vi "Inst.KH7008.AppLauncher.vi"(8 "error in":errorcluster, 11 "Debug Mode":bool) -> (0 "error out":errorcluster)   [LabVIEW 2019, in "Inst.KH7008.lvlib" / "Inst.Krohn-Hite-7008.lvclass"]
uses:
  Inst.Krohn-Hite-7008.lvclass
  Inst UI.Krohn-Hite-7008/Inst UI.Krohn-Hite-7008.lvclass
  <userlib>/LevyLab/Instrument Framework/Instrument/Instrument.lvclass
  <userlib>/LevyLab/Instrument Framework/Instrument UI/Instrument UI.lvclass
  <vilib>/JKI/JKI SMO/SMO/Typedefs/SMOState --Enum.ctl
  <vilib>/JKI/JKI SMO/SMO/SMO.lvclass
  <vilib>/JKI/JKI SMO/SMO.UI/SMO.UI.lvclass
  C:/Program Files/National Instruments/LabVIEW 2019/user.lib/LevyLab/Instrument Framework/Instrument Types/Amplifier/Instrument.Amplifier.lvclass
  C:/Program Files/National Instruments/LabVIEW 2019/user.lib/LevyLab/Instrument Framework/Instrument/Instrument.lvclass
  C:/Program Files/National Instruments/LabVIEW 2019/vi.lib/JKI/JKI SMO/SMO/SMO.lvclass
  C:/Program Files/National Instruments/LabVIEW 2019/user.lib/LevyLab/Instrument Framework/Instrument UI/Instrument UI.lvclass
  C:/Program Files/National Instruments/LabVIEW 2019/vi.lib/JKI/JKI SMO/SMO.UI/SMO.UI.lvclass
panel:
  in  "Examine Configuration.ini":bool
  in  "Splash Status":string="Push Start to Start..." caption="String"
  in  "Start Application":bool caption="Play"
  in  "Stop Application":bool caption="Stop"
  out "SMO State":T1
  # "Example Instrument SMO Test Launcher"
  # "For instructions on how to use the JKI State Machine Objects, examples and video tutorials, visit:\nhttp://jki.net/state-machine-objects/\n\nJKI State Machine Objects™\nhttp://jki.net/state-machine-objects/\nCopyright (C) 2005-2015, JKI <info@jki.net>\nALL RIGHTS RESERVED"
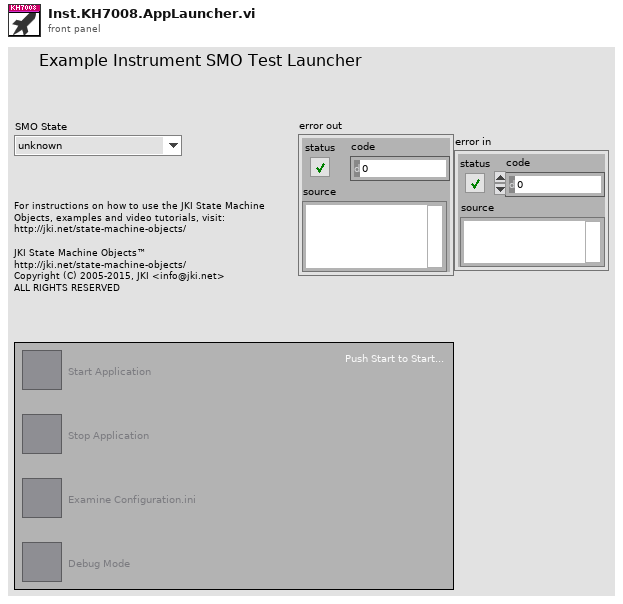
[diagram p1: front panel]
types:
  T1 = typedef "SMO.lvclass/SMOState --Enum.ctl" = enum16{"unknown", "Created", "Started", "Stopped"}
  T2 = enum32{"Invalid", "Standard", "Closed", "Hidden", "Minimized", "Maximized"}
  T3 = enum32{"invalid app kind", "Development System", "Run Time System", "Student Edition", "Embedded LabVIEW", "Evaluation", "Custom"}
  T4 = cluster{"Core":cluster{"Current VI Reference":refnum<vi>, "Close Panel on Exit?":bool}, "Instruments":refnum<class "Inst.Krohn-Hite-7008.lvclass">[], "Instrument UI":refnum<class "Inst UI.Krohn-Hite-7008.lvclass">[]}
  T5 = cluster{"Current VI Reference":refnum<vi>, "Close Panel on Exit?":bool}
  T6 = typedef "SMO.lvclass/Public Events.ctl" = cluster{"Error":refnum<user-event>, "State":refnum<user-event>, "Reserve State":refnum<user-event>}
  T7 = cluster{"Event Registration Refnum":refnum<event-registration>}
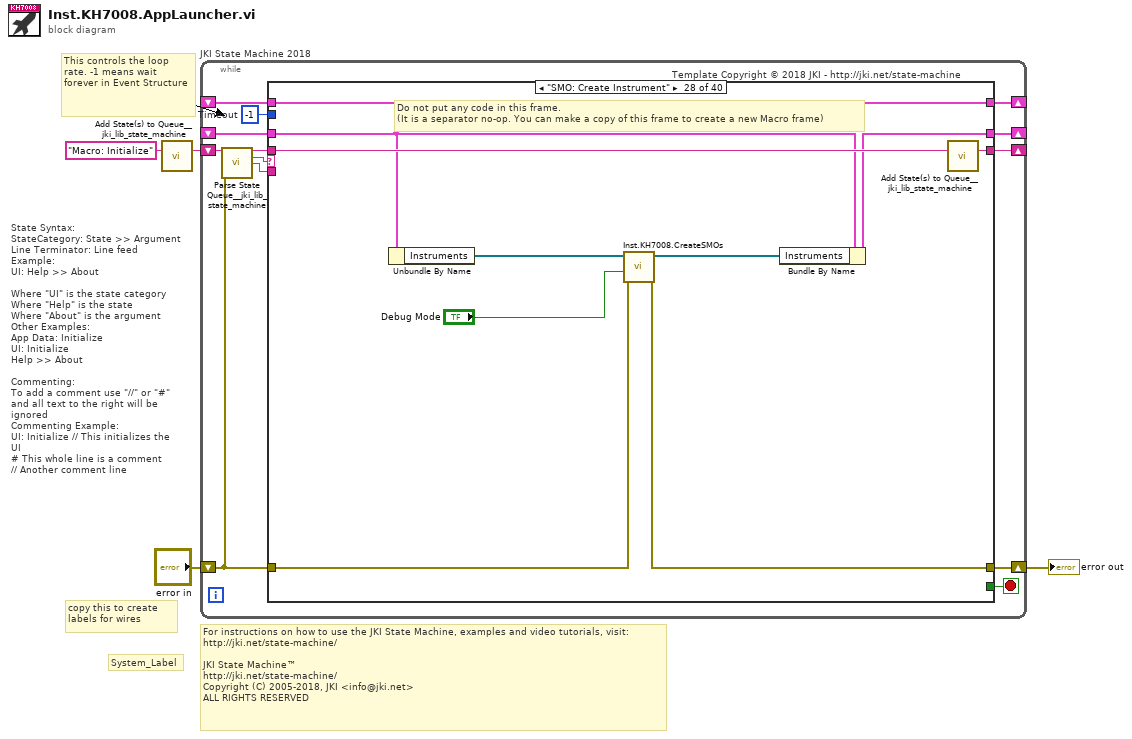
[diagram p0: block diagram]
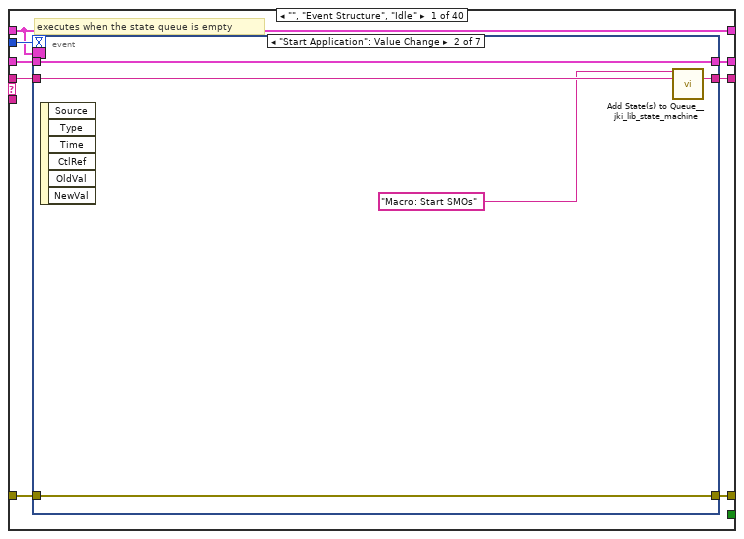
[diagram p2: hidden frame]
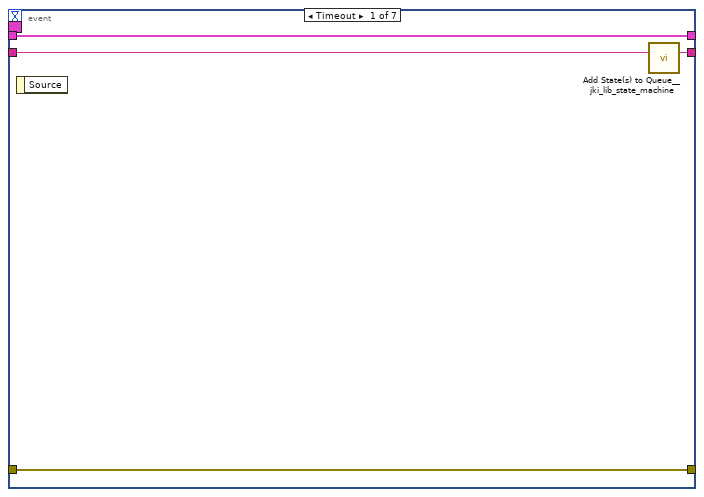
[diagram p3: hidden frame]
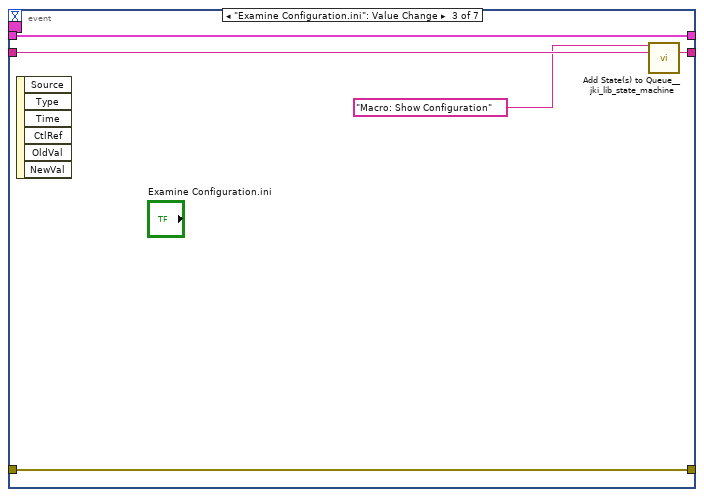
[diagram p4: hidden frame]
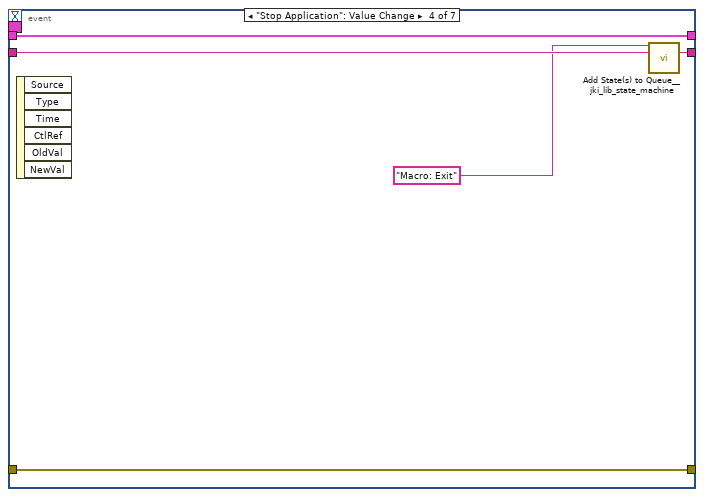
[diagram p5: hidden frame]
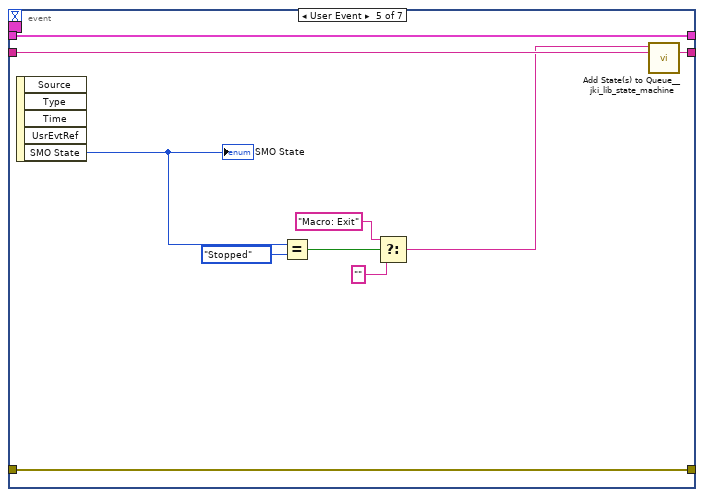
[diagram p6: hidden frame]
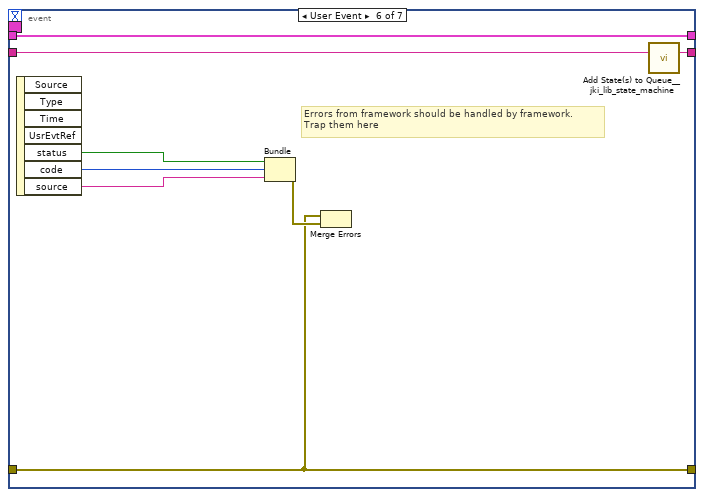
[diagram p7: hidden frame]
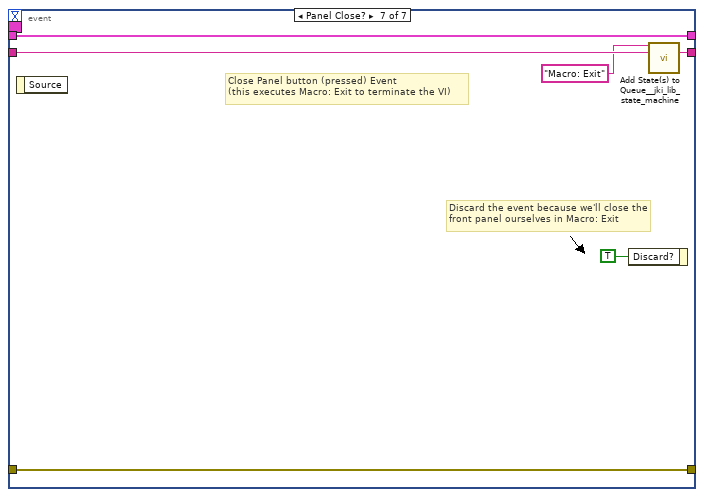
[diagram p8: hidden frame]
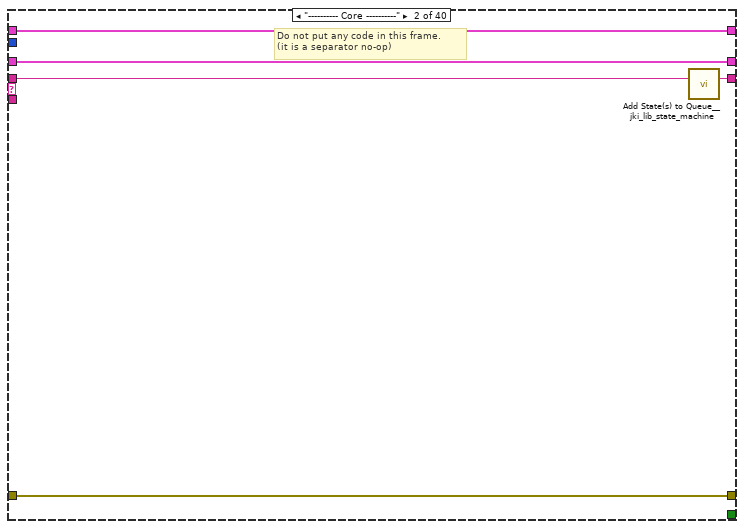
[diagram p9: hidden frame]
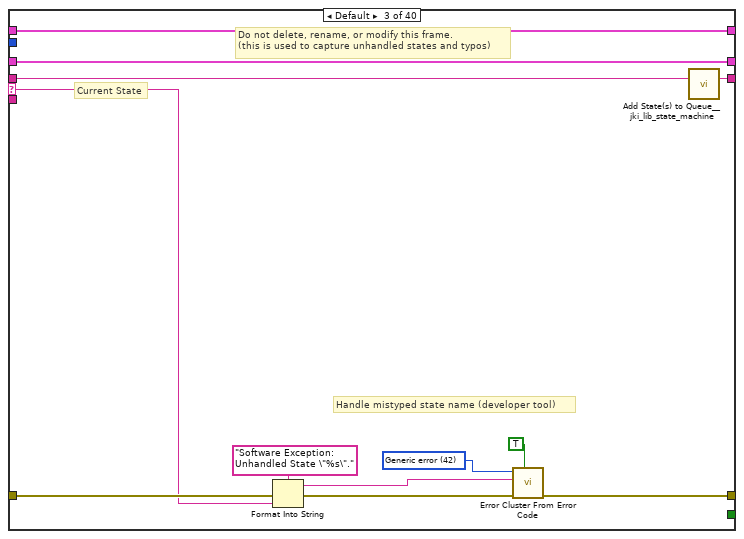
[diagram p10: hidden frame]
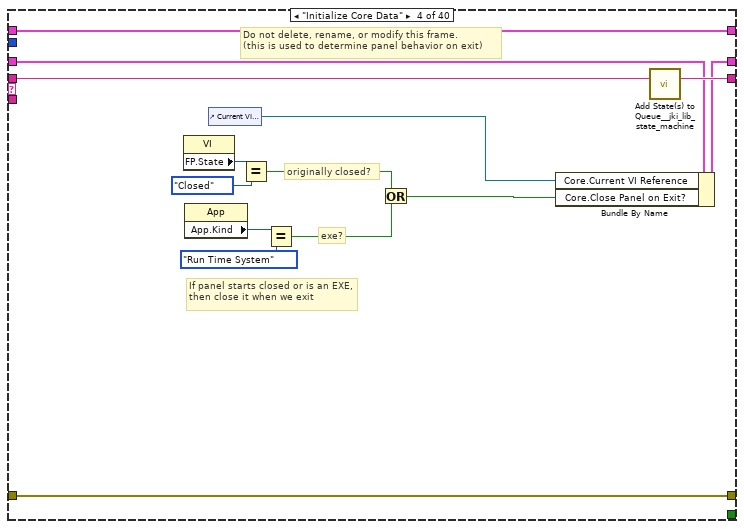
[diagram p11: hidden frame]
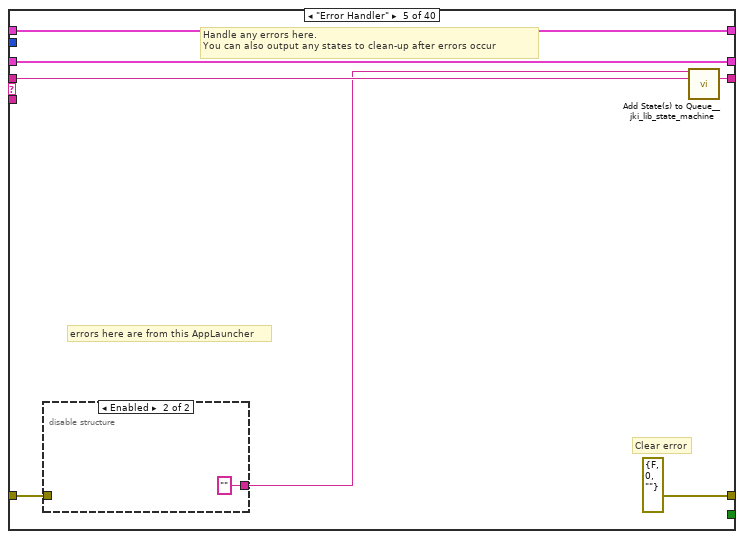
[diagram p12: hidden frame]
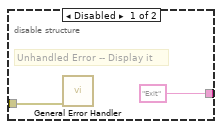
[diagram p13: hidden frame]
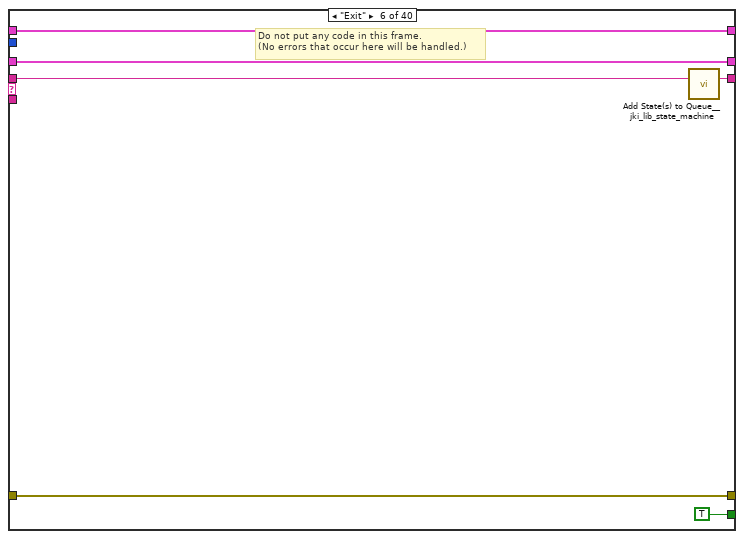
[diagram p14: hidden frame]
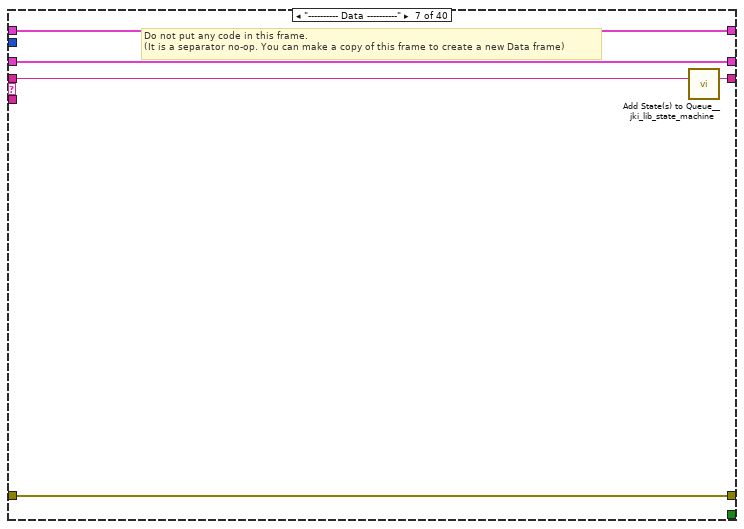
[diagram p15: hidden frame]
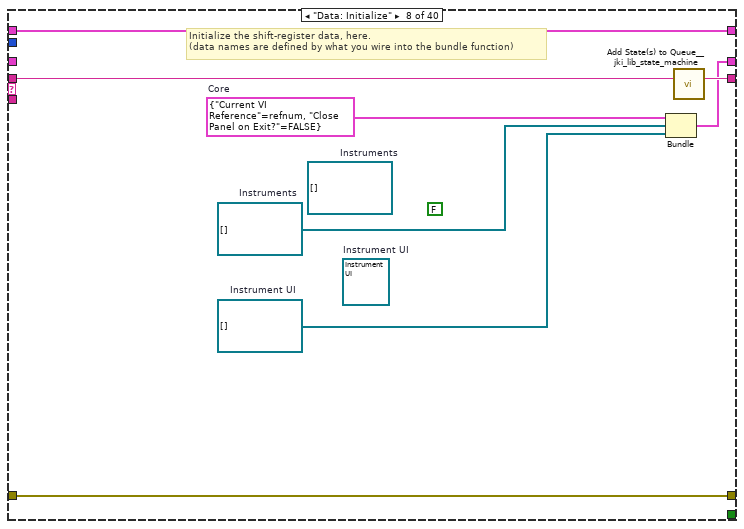
[diagram p16: hidden frame]
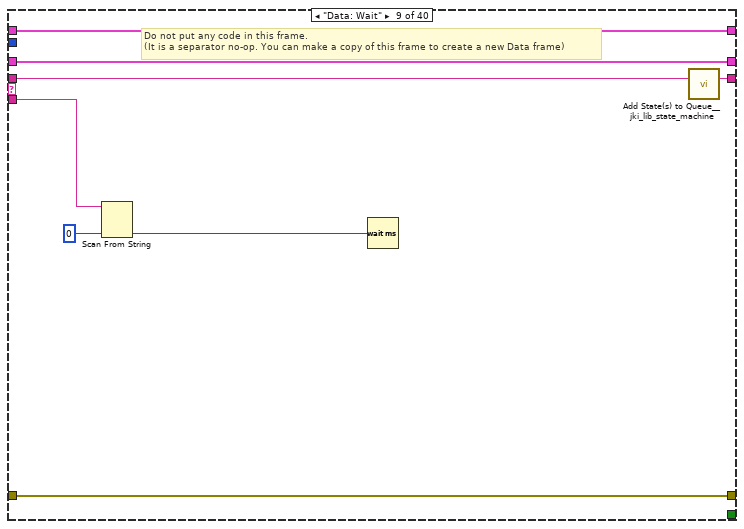
[diagram p17: hidden frame]
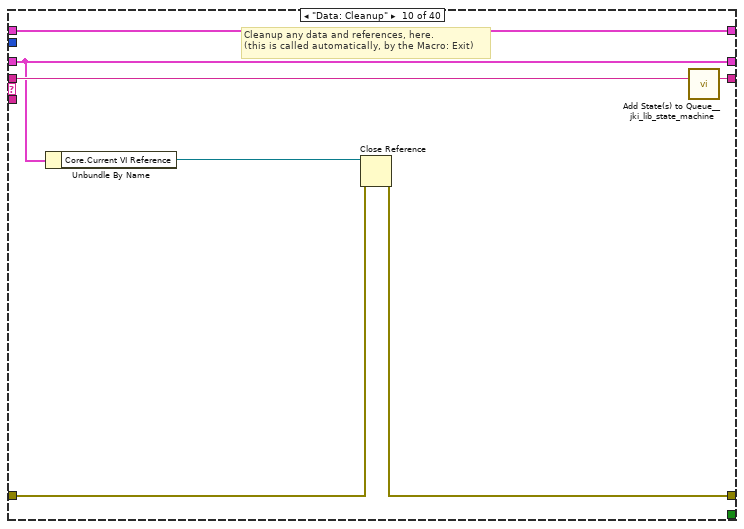
[diagram p18: hidden frame]
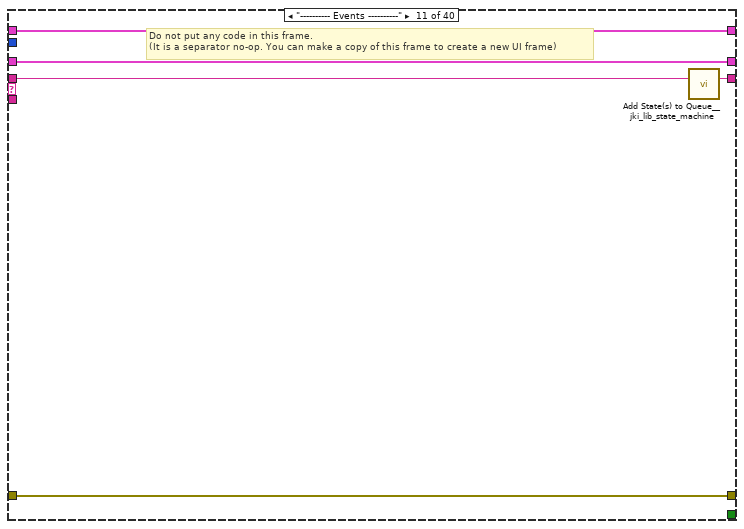
[diagram p19: hidden frame]
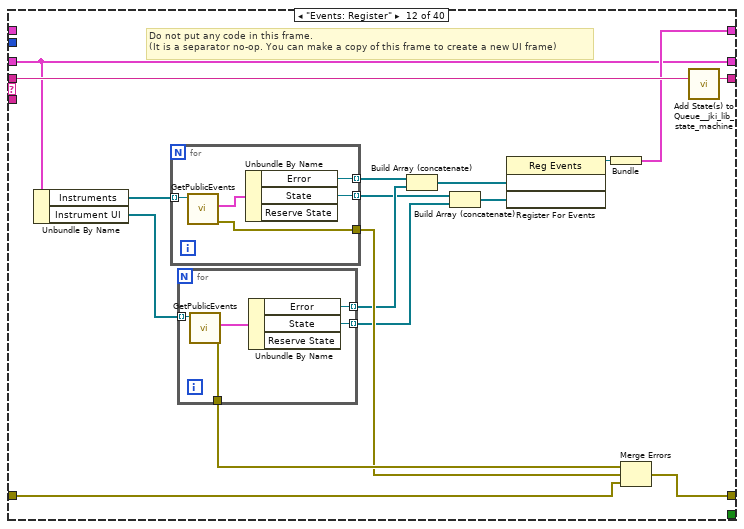
[diagram p20: hidden frame]
diagram:
  # "For instructions on how to use the JKI State Machine, examples and video tutorials, visit:\nhttp://jki.net/state-machine/\n\nJKI State Machine™\nhttp://jki.net/state-machine/\nCopyright (C) 2005-2018, JKI <info@jki.net>\nALL RIGHTS RESERVED"
  # "State Syntax:\nStateCategory: State >> Argument\nLine Terminator: Line feed\nExample:\nUI: Help >> About\n\nWhere \"UI\" is the state category\nWhere \"Help\" is the state\nWhere \"About\" is the argument\nOther Examples:\nApp Data: Initialize\nUI: Initialize\nHelp >> About\n\nCommenting:\nTo add a comment use \"//\" or \"#\" and all text to the right will be ignored\nCommenting Example:\nUI: Initialize // This initializes the UI\n# This whole line is a comment\n// Another comment line"
  # "copy this to create labels for wires"
  # "This controls the loop rate. -1 means wait forever in Event Structure"
  # "System_Label"
  n1 = call <vilib>:"Add State(s) to Queue__jki_lib_state_machine.vi"("State(s) in (\"\")"="Macro: Initialize") -> ("States Out"=w4:string)  [unwired: 14 in]
  n2 = while "JKI State Machine 2018" {
    shift-right: [w11] -> _
    shift-left: _ -> [w6]
    shift-right: [w14] -> w2
    shift-left: "error in" -> [w9]
    shift-right: [w13] -> _
    shift-left: w4 -> [w15]
    shift-right: [w8] -> _
    shift-left: _ -> [w7]
    stop <- w12 stop-if-true
    w10 = -1  # Timeout
    # "Template Copyright © 2018 JKI - http://jki.net/state-machine"
    n3 = call <vilib>:"Parse State Queue__jki_lib_state_machine.vi"("State Queue"=w15, "Error In (no error)"=w9) -> ("Remaining States"=w17:string, "Current State"=w5:string, "Arguments"=w16:string)  [unwired: 11 in]
    n4 = case shown="\"SMO: Create Instrument\"" w5 {
      selector: w5 -> [_ _ w75 _ _ _ _ _ _ _ _ _ _ _ _ _ _ _ _ _ _ _ _ _ _ _ _ _ _ _ _ _ _ _ _ _ _ _ _ _]
      tunnel: w17 -> [w25 w73 w79 w99 w106 w115 w120 w128 w136 w143 w148 w165 w181 w186 w193 w200 w212 w290 w297 w305 w310 w316 w322 w328 w334 w346 w351 w361 w370 w385 w397 w407 w425 w443 w461 w479 w497 w513 w520 w525]
      tunnel: w16 -> [_ _ _ _ _ _ _ _ w131 _ _ _ _ _ _ w195 w206 _ _ _ _ _ _ _ _ _ _ _ _ _ _ _ _ _ _ _ _ _ w517 _]
      tunnel: [w22 w71 w81 w96 errorcluster {"status"=FALSE, "code"=0, "source"=""} ("error out") w112 w118 w123 w134 w139 w146 w158 w177 w184 w188 w196 w209 w280 w294 w303 w308 w314 w320 w326 w332 w344 w349 w353 w362 w378 w391 w403 w421 w439 w458 w476 w494 w511 w515 w523] -> w14
      tunnel: w9 -> [w21 w71 w80 w96 w102 w112 w118 w123 w134 w140 w146 w157 w178 w184 w190 w197 w210 w281 w292 w303 w308 w314 w320 w326 w332 w344 w349 w354 w363 w379 w392 w402 w420 w438 w456 w474 w492 w511 w516 w523]
      tunnel: [w24 w72 w78 w98 w105 w114 w119 w127 w135 w142 w147 w164 w180 w185 w192 w199 w211 w289 w296 w304 w309 w315 w321 w327 w333 w345 w350 w360 w369 w384 w396 w406 w424 w442 w460 w478 w496 w512 w519 w524] -> w13
      tunnel: [_ _ _ _ _ TRUE _ _ _ _ _ _ _ _ _ _ _ _ _ _ _ _ _ _ _ _ _ _ _ _ _ _ _ _ _ _ _ _ _ _] -> w12
      tunnel: [w20 w70 w77 w97 w103 w113 w117 w126 w133 w138 w145 w162 w179 w183 w191 w198 w208 w278 w293 w302 w307 w313 w319 w325 w331 w343 w348 w358 w365 w381 w394 w404 w422 w440 w457 w475 w493 w510 w518 w522] -> w11
      tunnel: w10 -> [w19 _ _ _ _ _ _ _ _ _ _ _ _ _ _ _ _ _ _ _ _ _ _ _ _ _ _ _ _ _ _ _ _ _ _ _ _ _ _ _]
      tunnel: [w18 w69 w74 w86 w101 w110 w116 w124 w132 w137 w144 w163 w176 w182 w189 w194 w205 w279 w295 w301 w306 w311 w317 w324 w330 w337 w347 w359 w368 w383 w395 w405 w423 w441 w459 w477 w495 w509 w514 w521] -> w8
      tunnel: w7 -> [w18 w69 w74 w86 w101 w110 w116 w124 w132 w137 w144 _ w176 w182 w189 w194 w205 w279 w295 w301 w306 w311 w317 w324 w330 w337 w347 w359 w368 w383 w395 w405 w423 w441 w459 w477 w495 w509 w514 w521]
      tunnel: w6 -> [w23 w70 w77 w92 w103 w113 w117 _ w133 w138 w145 w162 w179 w183 w191 w198 w208 w278 w293 w302 w307 w313 w319 w325 w331 w343 w348 w356 w366 w382 w394 w404 w422 w440 w457 w475 w493 w510 w518 w522]
      frame "", "Event Structure", "Idle" {
        # "executes when the state queue is empty"
        n5 = event shown="[1] \"Start Application\": Value Change" {
          selector: w18 -> [_ _ _ _ _ _ _]
          dyn-events: _ -> [_ _ _ _ _ _ _]
          timeout: w19 -> [_ _ _ _ _ _ _]
          tunnel: w25 -> [w29 w34 w39 w44 w54 w62 w68]
          tunnel: [w28 w33 w38 w43 w53 w61 w67] -> w24
          tunnel: w23 -> [w26 w31 w36 w41 w51 w60 w65]
          tunnel: [w27 w32 w37 w42 w52 w55 w66] -> w22
          tunnel: w21 -> [w27 w32 w37 w42 w52 w55 w66]
          tunnel: [w26 w31 w36 w41 w51 w60 w65] -> w20
          event Timeout {
            n6 = event-data() -> ()  [unwired: 1 in, 1 out]
            n7 = call <vilib>:"Add State(s) to Queue__jki_lib_state_machine.vi"("State(s) in (\"\")"=w29) -> ("States Out"=w28:string)  [unwired: 14 in]
          }
          event "Start Application": Value Change {
            n8 = event-data() -> ()  [unwired: 1 in, 6 out]
            n9 = call <vilib>:"Add State(s) to Queue__jki_lib_state_machine.vi"("State(s) in Front (\"\")"="Macro: Start SMOs" ("State(s) in Front (\"\")"), "State(s) in (\"\")"=w34) -> ("States Out"=w33:string)  [unwired: 13 in]
          }
          event "Examine Configuration.ini": Value Change {
            n10 = event-data() -> ()  [unwired: 1 in, 6 out]
            n11 = call <vilib>:"Add State(s) to Queue__jki_lib_state_machine.vi"("State(s) in Front (\"\")"="Macro: Show Configuration" ("State(s) in Front (\"\")"), "State(s) in (\"\")"=w39) -> ("States Out"=w38:string)  [unwired: 13 in]
          }
          event "Stop Application": Value Change {
            n12 = event-data() -> ()  [unwired: 1 in, 6 out]
            n13 = call <vilib>:"Add State(s) to Queue__jki_lib_state_machine.vi"("State(s) in Front (\"\")"="Macro: Exit" ("State(s) in Front (\"\")"), "State(s) in (\"\")"=w44) -> ("States Out"=w43:string)  [unwired: 13 in]
          }
          event User Event {
            n14 = event-data() -> ("SMO State"=w46:T1)  [unwired: 1 in, 4 out]
            "SMO State" <- w46
            n15 = Equal?(x=w46, y=SMOState_--Enum."Stopped") -> (x = y?=w49:bool)
            n16 = Select(t="Macro: Exit", s=w49, f="" ("State(s) in Front (\"\")")) -> (s? t:f=w45:string)
            n17 = call <vilib>:"Add State(s) to Queue__jki_lib_state_machine.vi"("State(s) in Front (\"\")"=w45, "State(s) in (\"\")"=w54) -> ("States Out"=w53:string)  [unwired: 13 in]
          }
          event User Event {
            # "Errors from framework should be handled by framework.\nTrap them here"
            n18 = event-data() -> ("status"=w56:bool, "code"=w58:i32, "source"=w57:string)  [unwired: 1 in, 4 out]
            n19 = Bundle("status"=w56, "code"=w58, "source"=w57) -> (w59:errorcluster)  [unwired: 1 in]
            n20 = Merge Errors(w55, w59) -> ()  [unwired: 1 out]
            n21 = call <vilib>:"Add State(s) to Queue__jki_lib_state_machine.vi"("State(s) in (\"\")"=w62) -> ("States Out"=w61:string)  [unwired: 14 in]
          }
          event Panel Close? {
            # "Discard the event because we'll close the front panel ourselves in Macro: Exit"
            # "Close Panel button (pressed) Event\n(this executes Macro: Exit to terminate the VI)"
            n22 = event-data() -> ()  [unwired: 1 in, 1 out]
            n23 = event-data("Discard?"=TRUE) -> ()  [unwired: 1 in, 1 out]
            n24 = call <vilib>:"Add State(s) to Queue__jki_lib_state_machine.vi"("State(s) in Front (\"\")"="Macro: Exit", "State(s) in (\"\")"=w68) -> ("States Out"=w67:string)  [unwired: 13 in]
          }
        }
      }
      frame "---------- Core ----------" {
        # "Do not put any code in this frame.\n(it is a separator no-op)"
        n25 = call <vilib>:"Add State(s) to Queue__jki_lib_state_machine.vi"("State(s) in (\"\")"=w73) -> ("States Out"=w72:string)  [unwired: 14 in]
      }
      frame Default {
        w84 = 42 items=["No error", "Argument error", "Memory is full", "Out of zone", "End of file", "File already open", "Generic file I/O error", "File not found", "File permission error", "Disk is full", "Duplicate path", "Too many files open", "System feature not enabled", "Resource file not found", "Cannot add resource", "Resource not found", "Image not found", "Image memory error", "Pen does not exist", "Config type invalid", "Config token not found", "Config parse error", "Config memory error", "Bad external code format", "Bad external code offset", "External code not present", "Null window", "Destroy window error", "Null menu", "Print aborted", "Bad print record", "Print driver error", "Windows error during printing", "Memory error during printing", "Print dialog error", "Generic print error", "Invalid device refnum", "Device not found", "Device parameter error", "Device unit error", "Cannot open device", "Device call aborted", "Generic error", "Cancelled by user", "Object ID too low", "Object ID too high", "Object not in heap", "Unknown heap", "Unknown object (invalid DefProc)", "Unknown object (DefProc not in table)", "Message out of range", "Invalid (null) method", "Unknown message", "Manager call not supported", "Bad address", "Network operation in progress", "Network operation timed out", "Connection is busy", "Network attribute not supported", "Network error", "Address in use", "System out of memory", "Connection aborted", "Connection refused", "Not connected", "Already connected", "Connection closed", "Initialization error (interapplication manager)", "Bad occurrence", "Wait on unbound occurrence handler", "Occurrence queue overflow", "Datalog type conflict", "Unused", "Unrecognized type (interapplication manager)", "Memory corrupt", "Failed to make temporary DLL", "Old CIN version", "Drag socket not found", "Failed to load drop-object", "Failed to register OLE object", "Failed to release OLE object", "Format specifier type mismatch", "Unknown format specifier", "Too few format specifiers", "Too many format specifiers", "Scan failed", "Newer CIN version", "Error converting to variant", "Runtime menu error", "Password tampered", "Variant attribute not found", "Incompatible variant data type", "Event data is not available", "Event Store is not present", "Occurrence is not found", "Event Queue is not created", "Event info is not available", "Refnum passed is NULL", "Error retrieving Class GUID", "Error retrieving CoClass GUID", "Error retrieving TypeLib GUID.", "Bad built application magic bytes.", "Specific driver is different from the specific driver associated with the Logical Name.", "There is no session opened to the class driver.", "Max Error", "MAX - Error with config objects", "MAX - Error loading configuration", "MAX - Group not supported"]
        # "Current State"
        # "Do not delete, rename, or modify this frame.\n(this is used to capture unhandled states and typos)"
        # "Handle mistyped state name (developer tool)"
        n26 = Format Into String(format string="Software Exception: Unhandled State \"%s\"." ("message"), error in=w80, w75) -> (resulting string=w83:string, error out=w82:errorcluster)  [unwired: 1 in]
        n27 = call <vilib>:"Error Cluster From Error Code.vi"("show call chain? (False)"=TRUE, "error in (no error)"=w82, "error message (\"\")"=w83, "error code (0)"=w84) -> ("error out"=w81:errorcluster)  [unwired: 5 in]
        n28 = call <vilib>:"Add State(s) to Queue__jki_lib_state_machine.vi"("State(s) in (\"\")"=w79) -> ("States Out"=w78:string)  [unwired: 14 in]
      }
      frame "Initialize Core Data" {
        # "Do not delete, rename, or modify this frame.\n(this is used to determine panel behavior on exit)"
        # "originally closed?"
        # "exe?"
        # "If panel starts closed or is an EXE, then close it when we exit"
        n29 = property class="VI"() -> ("FP.State"=w89:T2)  [unwired: 2 in, 2 out]
        n30 = property class="App"() -> ("App.Kind"=w95:T3)  [unwired: 2 in, 2 out]
        n31 = control-ref of="Current VI Reference"() -> (w90:refnum<vi>)
        n32 = Equal?(x=w89, y=T2."Closed" ("Front Panel Window:State")) -> (x = y?=w87:bool)
        n33 = Equal?(x=w95, y=T3."Run Time System" ("Application:Kind")) -> (x = y?=w93:bool)
        n34 = Or(x=w87, y=w93) -> (x .or. y?=w91:bool)
        n35 = Bundle By Name(cluster=w92, "Core.Current VI Reference"=w90, "Core.Close Panel on Exit?"=w91) -> (w97:T4)
        n36 = call <vilib>:"Add State(s) to Queue__jki_lib_state_machine.vi"("State(s) in (\"\")"=w99) -> ("States Out"=w98:string)  [unwired: 14 in]
      }
      frame "Error Handler" {
        # "errors here are from this AppLauncher"
        # "Handle any errors here.\nYou can also output any states to clean-up after errors occur"
        # "Clear error"
        n37 = disable-structure shown="Enabled" {
          disable-tunnel: w102 -> [w108 _]
          disable-tunnel: ["Exit" "" ("State(s) in Front (\"\")")] -> w100
          frame Disabled {
            # "Unhandled Error -- Display it"
            n38 = call <vilib>:"General Error Handler.vi"("error in (no error)"=w108) -> ()  [unwired: 10 in, 5 out]
          }
          frame Enabled {
          }
        }
        n39 = call <vilib>:"Add State(s) to Queue__jki_lib_state_machine.vi"("State(s) in Front (\"\")"=w100, "State(s) in (\"\")"=w106) -> ("States Out"=w105:string)  [unwired: 13 in]
      }
      frame "Exit" {
        # "Do not put any code in this frame.\n(No errors that occur here will be handled.)"
        n40 = call <vilib>:"Add State(s) to Queue__jki_lib_state_machine.vi"("State(s) in (\"\")"=w115) -> ("States Out"=w114:string)  [unwired: 14 in]
      }
      frame "---------- Data ----------" {
        # "Do not put any code in this frame.\n(It is a separator no-op. You can make a copy of this frame to create a new Data frame)"
        n41 = call <vilib>:"Add State(s) to Queue__jki_lib_state_machine.vi"("State(s) in (\"\")"=w120) -> ("States Out"=w119:string)  [unwired: 14 in]
      }
      frame "Data: Initialize" {
        (unwired) FALSE ("s")
        w122 = refnum<class "Inst.Krohn-Hite-7008.lvclass">[] []  # Instruments
        w121 = refnum<class "Inst UI.Krohn-Hite-7008.lvclass">[] []  # Instrument UI
        (unwired) refnum<class "Instrument UI.lvclass"> refnum  # Instrument UI
        (unwired) refnum<class "Instrument.lvclass">[] []  # Instruments
        w125 = T5 {"Current VI Reference"=refnum, "Close Panel on Exit?"=FALSE}  # Core
        # "Initialize the shift-register data, here.\n(data names are defined by what you wire into the bundle function)"
        n42 = Bundle("Core"=w125, "Instruments"=w122, "Instrument UI"=w121) -> (w126:T4)  [unwired: 1 in]
        n43 = call <vilib>:"Add State(s) to Queue__jki_lib_state_machine.vi"("State(s) in (\"\")"=w128) -> ("States Out"=w127:string)  [unwired: 14 in]
      }
      frame "Data: Wait" {
        # "Do not put any code in this frame.\n(It is a separator no-op. You can make a copy of this frame to create a new Data frame)"
        n44 = Scan From String(input string=w131, default 1=u32 0) -> (output 1=w129:u32)  [unwired: 3 in, 3 out]
        n45 = Wait (ms)(milliseconds to wait=w129) -> ()  [unwired: 1 out]
        n46 = call <vilib>:"Add State(s) to Queue__jki_lib_state_machine.vi"("State(s) in (\"\")"=w136) -> ("States Out"=w135:string)  [unwired: 14 in]
      }
      frame "Data: Cleanup" {
        # "Cleanup any data and references, here.\n(this is called automatically, by the Macro: Exit)"
        n47 = Unbundle By Name(w138) -> ("Core.Current VI Reference"=w141:refnum<vi>)
        n48 = Close Reference(reference=w141, error in (no error)=w140) -> (error out=w139:errorcluster)
        n49 = call <vilib>:"Add State(s) to Queue__jki_lib_state_machine.vi"("State(s) in (\"\")"=w143) -> ("States Out"=w142:string)  [unwired: 14 in]
      }
      frame "---------- Events ----------" {
        # "Do not put any code in this frame.\n(It is a separator no-op. You can make a copy of this frame to create a new UI frame)"
        n50 = call <vilib>:"Add State(s) to Queue__jki_lib_state_machine.vi"("State(s) in (\"\")"=w148) -> ("States Out"=w147:string)  [unwired: 14 in]
      }
      frame "Events: Register" {
        # "Do not put any code in this frame.\n(It is a separator no-op. You can make a copy of this frame to create a new UI frame)"
        n51 = Unbundle By Name(w162) -> ("Instruments"=w161:refnum<class "Inst.Krohn-Hite-7008.lvclass">[], "Instrument UI"=w160:refnum<class "Inst UI.Krohn-Hite-7008.lvclass">[])
        n52 = for {
          tunnel: w161 -> [w175] mode=indexing
          tunnel: [w174] -> w155
          tunnel: [w172] -> w154 mode=indexing
          tunnel: [w171] -> w151 mode=indexing
          n53 = call <vilib>:"GetPublicEvents.vi"("SMO"=w175) -> ("error out"=w174:errorcluster, "Public Events"=w173:T6)  [unwired: 8 in, 1 out]
          n54 = Unbundle By Name(w173) -> ("Error"=w172:refnum<user-event>, "State"=w171:refnum<user-event>)  [unwired: 1 out]
        }
        n55 = for {
          tunnel: w160 -> [w170] mode=indexing
          tunnel: [w169] -> w159
          tunnel: [w167] -> w153 mode=indexing
          tunnel: [w166] -> w149 mode=indexing
          n56 = call <vilib>:"GetPublicEvents.vi"("SMO"=w170) -> ("error out"=w169:errorcluster, "Public Events"=w168:T6)  [unwired: 8 in, 1 out]
          n57 = Unbundle By Name(w168) -> ("Error"=w167:refnum<user-event>, "State"=w166:refnum<user-event>)  [unwired: 1 out]
        }
        n58 = Build Array (concatenate)(w154, w153) -> (w152:refnum<user-event>[])
        n59 = Build Array (concatenate)(w151, w149) -> (w150:refnum<user-event>[])
        n60 = register-events(w152, w150) -> (reference out=w156:refnum<event-registration>)  [unwired: 2 in, 1 out]
        n61 = Bundle("Event Registration Refnum"=w156) -> (w163:T7)  [unwired: 1 in]
        n62 = Merge Errors(w159, w155, w157) -> (w158:errorcluster)
        n63 = call <vilib>:"Add State(s) to Queue__jki_lib_state_machine.vi"("State(s) in (\"\")"=w165) -> ("States Out"=w164:string)  [unwired: 14 in]
      }
      frame "Events: Unregister" {
        # "Do not put any code in this frame.\n(It is a separator no-op. You can make a copy of this frame to create a new UI frame)"
        n64 = Unregister For Events(event registration refnum=w176, error in=w178) -> (error out=w177:errorcluster)
        n65 = call <vilib>:"Add State(s) to Queue__jki_lib_state_machine.vi"("State(s) in (\"\")"=w181) -> ("States Out"=w180:string)  [unwired: 14 in]
      }
      frame "---------- UI ----------" {
        # "Do not put any code in this frame.\n(It is a separator no-op. You can make a copy of this frame to create a new UI frame)"
        n66 = call <vilib>:"Add State(s) to Queue__jki_lib_state_machine.vi"("State(s) in (\"\")"=w186) -> ("States Out"=w185:string)  [unwired: 14 in]
      }
      frame "UI: Initialize" {
        # "Initialize the User Interface, here.\n(this is called automatically, by the Macro: Init)"
        n67 = invoke on="Stop Application" class="Bool" method="Reinit To Default"() -> ()  [unwired: 3 in, 3 out]
        n68 = invoke on="error out" class="Clust (strict)" method="Reinit To Default"() -> ()  [unwired: 3 in, 3 out]
        n69 = invoke on="SMO State" class="Enum (strict)" method="Reinit To Default"() -> ()  [unwired: 3 in, 3 out]
        n70 = invoke on="Start Application" class="Bool" method="Reinit To Default"() -> ()  [unwired: 3 in, 3 out]
        n71 = call <userlib>:"Fit VI window to Largest Dec__ogtk.vi"("error in (no error)"=w190, "border spacing (2 px)"=1) -> ("error out"=w188:errorcluster)  [unwired: 4 in, 1 out]
        n72 = call <vilib>:"Add State(s) to Queue__jki_lib_state_machine.vi"("State(s) in (\"\")"=w193) -> ("States Out"=w192:string)  [unwired: 14 in]
      }
      frame "UI: Cursor Set" {
        # "Argument"
        # "Set and Unset Cursor Busy.\n(Usage: \"UI: Cursor Set >> Busy|Idle\")"
        n73 = case shown="\"Busy\"" w195 {
          tunnel: w197 -> [w202 w204]
          tunnel: [w201 w203] -> w196
          frame "Idle", Default {
            n74 = call <vilib>:"Unset Busy.vi"("error in (no error)"=w202) -> ("error out"=w201:errorcluster)  [unwired: 10 in]
          }
          frame "Busy" {
            n75 = call <vilib>:"Set Busy.vi"("error in (no error)"=w204) -> ("error out"=w203:errorcluster)  [unwired: 9 in, 1 out]
          }
        }
        n76 = call <vilib>:"Add State(s) to Queue__jki_lib_state_machine.vi"("State(s) in (\"\")"=w200) -> ("States Out"=w199:string)  [unwired: 14 in]
      }
      frame "UI: Front Panel State" {
        # "Argument"
        # "Set Front Panel Open or Closed\n(Usage: \"UI: Front Panel State >> Open|Close\")"
        n77 = Unbundle By Name(w208) -> ("Core.Current VI Reference"=w207:refnum<vi>)
        n78 = case shown="\"Open\", \"Standard\", Default" w206 {
          tunnel: w210 -> [w218 w233 w244 w257 w270]
          tunnel: [w220 w234 w246 w259 w272] -> w209
          tunnel: w207 -> [w219 w231 w245 w258 w271]
          frame "Open", "Standard", Default {
            w213 = T2."Standard" ("State")
            n79 = property class="VI"(reference=w219, error in=w218) -> (reference out=w216:refnum<vi>, error out=w217:errorcluster, "FP.State"=w215:T2)
            n80 = Not Equal?(x=w215, y=w213) -> (x != y?=w214:bool)
            n81 = case shown="False" w214 {
              tunnel: [w224 w226] -> w220
              tunnel: w217 -> [w223 w226]
              tunnel: w216 -> [w222 _]
              tunnel: w213 -> [w221 _]
              frame True {
                n82 = invoke class="VI" method="FP.Open"(reference=w222, error in=w223, "Activate"=TRUE, "State"=w221) -> (error out=w224:errorcluster)  [unwired: 1 in, 4 out]
              }
              frame False {
              }
            }
          }
          frame "Close", "Closed" {
            n83 = property class="VI"(reference=w231, error in=w233) -> (reference out=w230:refnum<vi>, error out=w232:errorcluster, "FP.State"=w228:T2)
            n84 = Not Equal?(x=w228, y=T2."Closed" ("Front Panel Window:State")) -> (x != y?=w227:bool)
            n85 = case shown="True" w227 {
              tunnel: [w235 w238] -> w234
              tunnel: w232 -> [w235 w237]
              tunnel: w230 -> [_ w236]
              frame False {
              }
              frame True {
                n86 = invoke class="VI" method="FP.Close"(reference=w236, error in=w237) -> (error out=w238:errorcluster)  [unwired: 1 in, 2 out]
              }
            }
          }
          frame "Hidden", "Hide" {
            w239 = T2."Hidden" ("State")
            n87 = property class="VI"(reference=w245, error in=w244) -> (reference out=w242:refnum<vi>, error out=w243:errorcluster, "FP.State"=w241:T2)
            n88 = Not Equal?(x=w241, y=w239) -> (x != y?=w240:bool)
            n89 = case shown="True" w240 {
              tunnel: [w250 w251] -> w246
              tunnel: w243 -> [w249 w251]
              tunnel: w242 -> [w248 _]
              tunnel: w239 -> [w247 _]
              frame True {
                n90 = invoke class="VI" method="FP.Open"(reference=w248, error in=w249, "State"=w247) -> (error out=w250:errorcluster)  [unwired: 2 in, 4 out]
              }
              frame False {
              }
            }
          }
          frame "Minimize", "Minimized" {
            w252 = T2."Minimized" ("State")
            n91 = property class="VI"(reference=w258, error in=w257) -> (reference out=w255:refnum<vi>, error out=w256:errorcluster, "FP.State"=w254:T2)
            n92 = Not Equal?(x=w254, y=w252) -> (x != y?=w253:bool)
            n93 = case shown="True" w253 {
              tunnel: [w263 w264] -> w259
              tunnel: w256 -> [w262 w264]
              tunnel: w255 -> [w261 _]
              tunnel: w252 -> [w260 _]
              frame True {
                n94 = invoke class="VI" method="FP.Open"(reference=w261, error in=w262, "State"=w260) -> (error out=w263:errorcluster)  [unwired: 2 in, 4 out]
              }
              frame False {
              }
            }
          }
          frame "Maximize", "Maximized" {
            w265 = T2."Maximized" ("State")
            n95 = property class="VI"(reference=w271, error in=w270) -> (reference out=w268:refnum<vi>, error out=w269:errorcluster, "FP.State"=w267:T2)
            n96 = Not Equal?(x=w267, y=w265) -> (x != y?=w266:bool)
            n97 = case shown="True" w266 {
              tunnel: [w276 w277] -> w272
              tunnel: w269 -> [w275 w277]
              tunnel: w268 -> [w274 _]
              tunnel: w265 -> [w273 _]
              frame True {
                n98 = invoke class="VI" method="FP.Open"(reference=w274, error in=w275, "State"=w273) -> (error out=w276:errorcluster)  [unwired: 2 in, 4 out]
              }
              frame False {
              }
            }
          }
        }
        n99 = call <vilib>:"Add State(s) to Queue__jki_lib_state_machine.vi"("State(s) in (\"\")"=w212) -> ("States Out"=w211:string)  [unwired: 14 in]
      }
      frame "UI: Set Background Color" {
        # "Do not put any code in this frame.\n(It is a separator no-op. You can make a copy of this frame to create a new UI frame)"
        n100 = property class="VI"(error in=w281) -> (error out=w283:errorcluster, "Panel"=w284:refnum<vi>)  [unwired: 1 in, 1 out]
        n101 = property class="Pnl"(reference=w284, error in=w283) -> (error out=w282:errorcluster, "Panes[]"=w285:refnum<vi>[])  [unwired: 1 out]
        n102 = Index Array(array=w285, index=0) -> (element=w287:refnum<vi>)
        n103 = property class="Pane"(reference=w287, error in=w282, "PaneColor"=u32 16777238 ("Color Box")) -> (error out=w280:errorcluster)  [unwired: 1 out]
        n104 = call <vilib>:"Add State(s) to Queue__jki_lib_state_machine.vi"("State(s) in (\"\")"=w290) -> ("States Out"=w289:string)  [unwired: 14 in]
      }
      frame "UI: Open Configuration.ini" {
        # "Do not put any code in this frame.\n(It is a separator no-op. You can make a copy of this frame to create a new UI frame)"
        n105 = Unbundle By Name(w293) -> ("Instruments"=w291:refnum<class "Inst.Krohn-Hite-7008.lvclass">[])
        n106 = for {
          shift-right: [w300] -> w294
          shift-left: w292 -> [w299]
          tunnel: w291 -> [w298] mode=indexing
          n107 = call <userlib>:"Examine Configuration.vi"("error in (no error)"=w299, "Instrument in"=w298) -> ("error out"=w300:errorcluster)  [unwired: 8 in, 1 out]
        }
        n108 = call <vilib>:"Add State(s) to Queue__jki_lib_state_machine.vi"("State(s) in (\"\")"=w297) -> ("States Out"=w296:string)  [unwired: 14 in]
      }
      frame "UI: Exit" {
        # "Do not put any code in this frame.\n(It is a separator no-op. You can make a copy of this frame to create a new UI frame)"
        n109 = invoke on="Start Application" class="Bool" method="Reinit To Default"() -> ()  [unwired: 3 in, 3 out]
        n110 = invoke on="Stop Application" class="Bool" method="Reinit To Default"() -> ()  [unwired: 3 in, 3 out]
        n111 = call <vilib>:"Add State(s) to Queue__jki_lib_state_machine.vi"("State(s) in (\"\")"=w305) -> ("States Out"=w304:string)  [unwired: 14 in]
      }
      frame "---------- Macro ----------" {
        # "Do not put any code in this frame.\n(It is a separator no-op. You can make a copy of this frame to create a new Macro frame)"
        n112 = call <vilib>:"Add State(s) to Queue__jki_lib_state_machine.vi"("State(s) in (\"\")"=w310) -> ("States Out"=w309:string)  [unwired: 14 in]
      }
      frame "Macro: Initialize" {
        # "Initialization Macro\n(This is called once, when the VI starts)"
        n113 = call <vilib>:"Add State(s) to Queue__jki_lib_state_machine.vi"("State(s) in Front (\"\")"="Data: Initialize\nInitialize Core Data\n//Events: Register\nUI: Initialize\nUI: Front Panel State >> Open\nUI: Set Background Color\nSplash: Set Status >> ...", "State(s) in (\"\")"=w316) -> ("States Out"=w315:string)  [unwired: 13 in]
      }
      frame "Macro: Show Configuration" {
        # "Initialization Macro\n(This is called once, when the VI starts)"
        n114 = call <vilib>:"Add State(s) to Queue__jki_lib_state_machine.vi"("State(s) in Front (\"\")"="Splash: Set Status >> Opeing Configuration...\nUI: Open Configuration.ini\nData: Wait >> 1000\nSplash: Set Status >> ...", "State(s) in (\"\")"=w322) -> ("States Out"=w321:string)  [unwired: 13 in]
      }
      frame "Macro: Start SMOs" {
        # "Do not put any code in this frame.\n(It is a separator no-op. You can make a copy of this frame to create a new Macro frame)"
        n115 = call <vilib>:"Add State(s) to Queue__jki_lib_state_machine.vi"("State(s) in Front (\"\")"="Splash: Set Status >> Creating Instrument...\nSMO: Create Instrument\nData: Wait >> 100\nSplash: Set Status >> Creating Instrument UI...\nSMO: Create Instrument UI\nData: Wait >> 100\nSplash: Set Status >> Registering Events...\nEvents: Register\nData: Wait >> 100\nSplash: Set Status >> Starting Instrument...\nSMO: Start Instrument\nData: Wait >> 100\nSplash: Set Status >> Instrument Process Started...\nData: Wait >> 100\nSplash: Set Status >> Starting User Interface...\nSMO: Start Instrument UI\nData: Wait >> 100\nUI: Front Panel State >> Hide\nSMO: Show Instrument UI" ("State(s) in Front (\"\")"), "State(s) in (\"\")"=w328) -> ("States Out"=w327:string)  [unwired: 13 in]
      }
      frame "Macro: Stop SMOs" {
        # "#todo\nshould stopping UI go before stopping Instrument?"
        # "Do not put any code in this frame.\n(It is a separator no-op. You can make a copy of this frame to create a new Macro frame)"
        n116 = call <vilib>:"Add State(s) to Queue__jki_lib_state_machine.vi"("State(s) in Front (\"\")"="UI: Front Panel State >> Show\nSplash: Set Status >> Stopping Instrument...\nSMO: Stop Instrument\nData: Wait >> 100\nSplash: Set Status >> Destroying Instrument...\nSMO: Destroy Instrument\nData: Wait >> 100\nSplash: Set Status >>Hiding UI...\nSMO: Hide Instrument UI\nData: Wait >> 100\nSplash: Set Status >> Stopping UI...\nSMO: Stop Instrument UI\nData: Wait >> 100\nSplash: Set Status >> Destroying UI...\nSMO: Destroy Instrument UI" ("State(s) in Front (\"\")"), "State(s) in (\"\")"=w334) -> ("States Out"=w333:string)  [unwired: 13 in]
      }
      frame "Macro: Exit" {
        # "Exit Macro\n(This is called once, when the VI exits)"
        n117 = Unbundle By Name(w343) -> ("Core.Close Panel on Exit?"=w342:bool)
        n118 = Select(t="UI: Front Panel State >> Close", s=w342, f="" ("Empty String Constant")) -> (s? t:f=w339:string)
        n119 = call <vilib>:"Add State(s) to Queue__jki_lib_state_machine.vi"("State(s) in Front (\"\")"="UI: Front Panel State >> Open\nUI: Exit\nMacro: Stop SMOs", "State(s) in (\"\")"=w339, "State(s) at Back (\"\")"="Data: Cleanup\nEvents: Unregister\nExit") -> ("States Out"=w338:string)  [unwired: 12 in]
        n120 = call <vilib>:"Add State(s) to Queue__jki_lib_state_machine.vi"("State(s) in Front (\"\")"=w338, "State(s) in (\"\")"=w346) -> ("States Out"=w345:string)  [unwired: 13 in]
      }
      frame "---------- SMO ----------" {
        # "Do not put any code in this frame.\n(It is a separator no-op. You can make a copy of this frame to create a new Macro frame)"
        n121 = call <vilib>:"Add State(s) to Queue__jki_lib_state_machine.vi"("State(s) in (\"\")"=w351) -> ("States Out"=w350:string)  [unwired: 14 in]
      }
      frame "SMO: Create Instrument" {
        # "Do not put any code in this frame.\n(It is a separator no-op. You can make a copy of this frame to create a new Macro frame)"
        n122 = Unbundle By Name(w356) -> ("Instruments"=w355:refnum<class "Inst.Krohn-Hite-7008.lvclass">[])
        n123 = call "Inst.KH7008.CreateSMOs.vi"("error in (no error)"=w354, "Debug Mode"="Debug Mode", "Instruments"=w355) -> ("error out"=w353:errorcluster, "Instruments out"=w357:refnum<class "Inst.Krohn-Hite-7008.lvclass">[])  [unwired: 7 in]
        n124 = Bundle By Name(cluster=w356, "Instruments"=w357) -> (w358:T4)
        n125 = call <vilib>:"Add State(s) to Queue__jki_lib_state_machine.vi"("State(s) in (\"\")"=w361) -> ("States Out"=w360:string)  [unwired: 14 in]
      }
      frame "SMO: Start Instrument" {
        # "Do not put any code in this frame.\n(It is a separator no-op. You can make a copy of this frame to create a new Macro frame)"
        n126 = Unbundle By Name(w366) -> ("Instruments"=w367:refnum<class "Inst.Krohn-Hite-7008.lvclass">[])
        n127 = for {
          tunnel: w367 -> [w374] mode=indexing
          tunnel: [w373] -> w364 mode=indexing
          tunnel: w363 -> [w372]
          tunnel: [w371] -> w362
          n128 = call <vilib>:"Start.vi"("error in (no error)"=w372, "SMO"=w374) -> ("error out"=w371:errorcluster, "SMO out"=w373:refnum<class "Inst.Krohn-Hite-7008.lvclass">)  [unwired: 8 in]
        }
        n129 = Bundle By Name(cluster=w366, "Instruments"=w364) -> (w365:T4)
        n130 = call <vilib>:"Add State(s) to Queue__jki_lib_state_machine.vi"("State(s) in (\"\")"=w370) -> ("States Out"=w369:string)  [unwired: 14 in]
      }
      frame "SMO: Create Instrument UI" {
        # "Do not put any code in this frame.\n(It is a separator no-op. You can make a copy of this frame to create a new Macro frame)"
        n131 = Unbundle By Name(w382) -> ("Instrument UI"=w376:refnum<class "Inst UI.Krohn-Hite-7008.lvclass">[], "Instruments"=w377:refnum<class "Inst.Krohn-Hite-7008.lvclass">[])
        n132 = Index Array(array=w376) -> (element=w375:refnum<class "Inst UI.Krohn-Hite-7008.lvclass">)  [unwired: 1 in]
        n133 = for {
          tunnel: w375 -> [w390]
          tunnel: w377 -> [w389] mode=indexing
          tunnel: [w387] -> w380 mode=indexing
          tunnel: w379 -> [w386]
          tunnel: [w388] -> w378
          n134 = call <userlib>:"Create UI.vi"("error in (no error)"=w386, "Instrument in"=w389, "Instrument UI"=w390) -> ("error out"=w388:errorcluster, "Instrument UI out"=w387:refnum<class "Inst UI.Krohn-Hite-7008.lvclass">)  [unwired: 7 in]
        }
        n135 = Bundle By Name(cluster=w382, "Instrument UI"=w380) -> (w381:T4)
        n136 = call <vilib>:"Add State(s) to Queue__jki_lib_state_machine.vi"("State(s) in (\"\")"=w385) -> ("States Out"=w384:string)  [unwired: 14 in]
      }
      frame "SMO: Start Instrument UI" {
        # "Do not put any code in this frame.\n(It is a separator no-op. You can make a copy of this frame to create a new Macro frame)"
        n137 = Unbundle By Name(w394) -> ("Instrument UI"=w393:refnum<class "Inst UI.Krohn-Hite-7008.lvclass">[])
        n138 = for {
          tunnel: w393 -> [w400] mode=indexing
          tunnel: w392 -> [w399]
          tunnel: [w398] -> w391
          n139 = call <vilib>:"Start.vi"("error in (no error)"=w399, "SMO"=w400) -> ("error out"=w398:errorcluster)  [unwired: 8 in, 1 out]
        }
        n140 = call <vilib>:"Add State(s) to Queue__jki_lib_state_machine.vi"("State(s) in (\"\")"=w397) -> ("States Out"=w396:string)  [unwired: 14 in]
      }
      frame "SMO: Show Instrument UI" {
        # "Do not put any code in this frame.\n(It is a separator no-op. You can make a copy of this frame to create a new Macro frame)"
        n141 = Unbundle By Name(w404) -> ("Instrument UI"=w401:refnum<class "Inst UI.Krohn-Hite-7008.lvclass">[])
        n142 = for {
          tunnel: w401 -> [w409] mode=indexing
          tunnel: w402 -> [w408]
          tunnel: [w414] -> w403
          n143 = call <vilib>:"GetState.vi"("error in (no error)"=w408, "SMO"=w409) -> ("error out"=w411:errorcluster, "SMO State"=w410:T1, "SMO out"=w413:refnum<class "Inst UI.Krohn-Hite-7008.lvclass">)  [unwired: 7 in]
          n144 = call <vilib>:"Clear Errors.vi"("error in (no error)"=w411) -> ("error out"=w412:errorcluster)  [unwired: 5 in, 1 out]
          n145 = case shown="\"Started\"" w410 {
            tunnel: [w415 w418] -> w414
            tunnel: w413 -> [_ w416]
            tunnel: w412 -> [w415 w417]
            frame Default {
            }
            frame "Started" {
              n146 = call <vilib>:"Show.vi"("error in (no error)"=w417, "SMO.UI"=w416) -> ("error out"=w418:errorcluster)  [unwired: 8 in, 1 out]
            }
          }
        }
        n147 = call <vilib>:"Add State(s) to Queue__jki_lib_state_machine.vi"("State(s) in (\"\")"=w407) -> ("States Out"=w406:string)  [unwired: 14 in]
      }
      frame "SMO: Destroy Instrument" {
        # "Do not put any code in this frame.\n(It is a separator no-op. You can make a copy of this frame to create a new Macro frame)"
        n148 = Unbundle By Name(w422) -> ("Instruments"=w419:refnum<class "Inst.Krohn-Hite-7008.lvclass">[])
        n149 = for {
          tunnel: w419 -> [w427] mode=indexing
          tunnel: w420 -> [w426]
          tunnel: [w432] -> w421
          n150 = call <vilib>:"GetState.vi"("error in (no error)"=w426, "SMO"=w427) -> ("error out"=w429:errorcluster, "SMO State"=w431:T1, "SMO out"=w428:refnum<class "Inst.Krohn-Hite-7008.lvclass">)  [unwired: 7 in]
          n151 = call <vilib>:"Clear Errors.vi"("error in (no error)"=w429) -> ("error out"=w430:errorcluster)  [unwired: 5 in, 1 out]
          n152 = case shown="\"Stopped\"" w431 {
            tunnel: [w433 w436] -> w432
            tunnel: w430 -> [w433 w435]
            tunnel: w428 -> [_ w434]
            frame Default {
            }
            frame "Stopped" {
              n153 = call <vilib>:"Destroy.vi"("error in (no error)"=w435, "SMO"=w434) -> ("error out"=w436:errorcluster)  [unwired: 9 in]
            }
          }
        }
        n154 = call <vilib>:"Add State(s) to Queue__jki_lib_state_machine.vi"("State(s) in (\"\")"=w425) -> ("States Out"=w424:string)  [unwired: 14 in]
      }
      frame "SMO: Hide Instrument UI" {
        # "Do not put any code in this frame.\n(It is a separator no-op. You can make a copy of this frame to create a new Macro frame)"
        n155 = Unbundle By Name(w440) -> ("Instrument UI"=w437:refnum<class "Inst UI.Krohn-Hite-7008.lvclass">[])
        n156 = for {
          tunnel: w437 -> [w445] mode=indexing
          tunnel: w438 -> [w444]
          tunnel: [w450] -> w439
          n157 = call <vilib>:"GetState.vi"("error in (no error)"=w444, "SMO"=w445) -> ("error out"=w447:errorcluster, "SMO State"=w446:T1, "SMO out"=w449:refnum<class "Inst UI.Krohn-Hite-7008.lvclass">)  [unwired: 7 in]
          n158 = call <vilib>:"Clear Errors.vi"("error in (no error)"=w447) -> ("error out"=w448:errorcluster)  [unwired: 5 in, 1 out]
          n159 = case shown="\"Started\"" w446 {
            tunnel: [w451 w454] -> w450
            tunnel: w449 -> [_ w452]
            tunnel: w448 -> [w451 w453]
            frame Default {
            }
            frame "Started" {
              n160 = call <vilib>:"Hide.vi"("error in (no error)"=w453, "SMO.UI"=w452) -> ("error out"=w454:errorcluster)  [unwired: 8 in, 1 out]
            }
          }
        }
        n161 = call <vilib>:"Add State(s) to Queue__jki_lib_state_machine.vi"("State(s) in (\"\")"=w443) -> ("States Out"=w442:string)  [unwired: 14 in]
      }
      frame "SMO: Stop Instrument UI" {
        # "Do not put any code in this frame.\n(It is a separator no-op. You can make a copy of this frame to create a new Macro frame)"
        n162 = Unbundle By Name(w457) -> ("Instrument UI"=w455:refnum<class "Inst UI.Krohn-Hite-7008.lvclass">[])
        n163 = for {
          tunnel: w455 -> [w463] mode=indexing
          tunnel: w456 -> [w462]
          tunnel: [w468] -> w458
          n164 = call <vilib>:"GetState.vi"("error in (no error)"=w462, "SMO"=w463) -> ("error out"=w467:errorcluster, "SMO State"=w465:T1, "SMO out"=w464:refnum<class "Inst UI.Krohn-Hite-7008.lvclass">)  [unwired: 7 in]
          n165 = call <vilib>:"Clear Errors.vi"("error in (no error)"=w467) -> ("error out"=w466:errorcluster)  [unwired: 5 in, 1 out]
          n166 = case shown="\"Created\", \"Started\"" w465 {
            tunnel: [w469 w472] -> w468
            tunnel: w464 -> [_ w471]
            tunnel: w466 -> [w469 w470]
            frame Default {
            }
            frame "Created", "Started" {
              n167 = call <vilib>:"Stop.vi"("error in (no error)"=w470, "SMO"=w471) -> ("error out"=w472:errorcluster)  [unwired: 8 in, 1 out]
            }
          }
        }
        n168 = call <vilib>:"Add State(s) to Queue__jki_lib_state_machine.vi"("State(s) in (\"\")"=w461) -> ("States Out"=w460:string)  [unwired: 14 in]
      }
      frame "SMO: Stop Instrument" {
        # "Do not put any code in this frame.\n(It is a separator no-op. You can make a copy of this frame to create a new Macro frame)"
        n169 = Unbundle By Name(w475) -> ("Instruments"=w473:refnum<class "Inst.Krohn-Hite-7008.lvclass">[])
        n170 = for {
          tunnel: w473 -> [w482] mode=indexing
          tunnel: w474 -> [w480]
          tunnel: [w486] -> w476
          n171 = call <vilib>:"GetState.vi"("error in (no error)"=w480, "SMO"=w482) -> ("error out"=w485:errorcluster, "SMO State"=w483:T1, "SMO out"=w481:refnum<class "Inst.Krohn-Hite-7008.lvclass">)  [unwired: 7 in]
          n172 = call <vilib>:"Clear Errors.vi"("error in (no error)"=w485) -> ("error out"=w484:errorcluster)  [unwired: 5 in, 1 out]
          n173 = case shown="\"Created\", \"Started\"" w483 {
            tunnel: [w487 w490] -> w486
            tunnel: w481 -> [_ w489]
            tunnel: w484 -> [w487 w488]
            frame Default {
            }
            frame "Created", "Started" {
              n174 = call <vilib>:"Stop.vi"("error in (no error)"=w488, "SMO"=w489) -> ("error out"=w490:errorcluster)  [unwired: 8 in, 1 out]
            }
          }
        }
        n175 = call <vilib>:"Add State(s) to Queue__jki_lib_state_machine.vi"("State(s) in (\"\")"=w479) -> ("States Out"=w478:string)  [unwired: 14 in]
      }
      frame "SMO: Destroy Instrument UI" {
        # "Do not put any code in this frame.\n(It is a separator no-op. You can make a copy of this frame to create a new Macro frame)"
        n176 = Unbundle By Name(w493) -> ("Instrument UI"=w491:refnum<class "Inst UI.Krohn-Hite-7008.lvclass">[])
        n177 = for {
          tunnel: w491 -> [w499] mode=indexing
          tunnel: w492 -> [w498]
          tunnel: [w504] -> w494
          n178 = call <vilib>:"GetState.vi"("error in (no error)"=w498, "SMO"=w499) -> ("error out"=w502:errorcluster, "SMO State"=w500:T1, "SMO out"=w503:refnum<class "Inst UI.Krohn-Hite-7008.lvclass">)  [unwired: 7 in]
          n179 = call <vilib>:"Clear Errors.vi"("error in (no error)"=w502) -> ("error out"=w501:errorcluster)  [unwired: 5 in, 1 out]
          n180 = case shown="\"Stopped\"" w500 {
            tunnel: w501 -> [w505 w508]
            tunnel: [w505 w507] -> w504
            tunnel: w503 -> [_ w506]
            frame Default {
            }
            frame "Stopped" {
              n181 = call <vilib>:"Destroy.vi"("error in (no error)"=w508, "SMO"=w506) -> ("error out"=w507:errorcluster)  [unwired: 9 in]
            }
          }
        }
        n182 = call <vilib>:"Add State(s) to Queue__jki_lib_state_machine.vi"("State(s) in (\"\")"=w497) -> ("States Out"=w496:string)  [unwired: 14 in]
      }
      frame "---------- Splash ----------" {
        # "Template Separator\n(You can make a copy of, or modify, this frame)"
        n183 = call <vilib>:"Add State(s) to Queue__jki_lib_state_machine.vi"("State(s) in (\"\")"=w513) -> ("States Out"=w512:string)  [unwired: 14 in]
      }
      frame "Splash: Set Status" {
        # "Your code here.\n(You can make a copy of, or modify, this frame)"
        n184 = property on="Splash Status" class="Str"(error in=w516, "Value"=w517) -> (error out=w515:errorcluster)  [unwired: 1 in, 1 out]
        n185 = call <vilib>:"Add State(s) to Queue__jki_lib_state_machine.vi"("State(s) in (\"\")"=w520) -> ("States Out"=w519:string)  [unwired: 14 in]
      }
      frame "Splash: 2" {
        # "Your code here.\n(You can make a copy of, or modify, this frame)"
        n186 = call <vilib>:"Add State(s) to Queue__jki_lib_state_machine.vi"("State(s) in (\"\")"=w525) -> ("States Out"=w524:string)  [unwired: 14 in]
      }
    }
  }
  "error out" <- w2
